vi "close-cam-session-if-exists.vi"(8 "error in (no error)":errorcluster, 11 "cam in":T1) -> (0 "error out":errorcluster)   [LabVIEW 2024]
uses:
  <vilib>/userDefined/High Color/IMAQdx.ctl
  <vilib>/vision/driver/NI_Vision_Acquisition_Software.lvlib
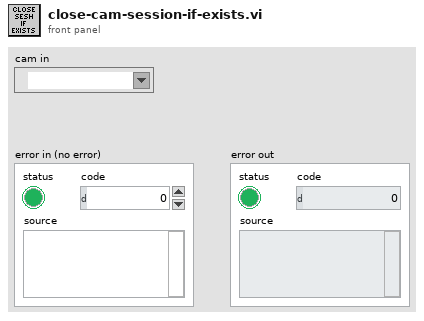
[diagram p1: front panel]
types:
  T1 = typedef "IMAQdx.ctl" = refnum<k21>
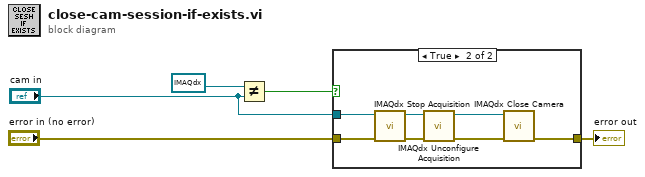
[diagram p0: block diagram]
diagram:
  n1 = Not Equal?(x=T1 refnum, y="cam in") -> (x != y?=w5:bool)
  n2 = case shown="True" w5 {
    tunnel: "error in (no error)" -> [w6 w10]
    tunnel: [w6 w13] -> w2
    tunnel: "cam in" -> [_ w11]
    frame False {
    }
    frame True {
      n3 = call <vilib>:"IMAQdx Stop Acquisition.vi"("error in"=w10, "Session In"=w11) -> ("error out"=w9:errorcluster, "Session Out"=w12:T1)  [unwired: 8 out]
      n4 = call <vilib>:"IMAQdx Unconfigure Acquisition.vi"("error in"=w9, "Session In"=w12) -> ("error out"=w8:errorcluster, "Session Out"=w7:T1)  [unwired: 8 out]
      n5 = call <vilib>:"IMAQdx Close Camera.vi"("error in"=w8, "Session In"=w7) -> ("error out"=w13:errorcluster)  [unwired: 9 out]
    }
  }
  "error out" <- w2
